vi "He3ReadOut_gpib.vi"(11 "reference":refnum<vi>) -> ()   [LabVIEW 2019]
uses:
  <vilib>/Utility/config.llb/Read Key (String).vi
  <vilib>/Utility/config.llb/NI_LVConfig.lvlib
panel:
  out "Last Updated":timestamp format="%<%Y-%m-%d %H:%M:%S>T"
  out "Device Version":dbl
  out "error out 4":errorcluster
  out "Pressure":waveform(dbl)[](graph)
  out "error out 3":errorcluster
  out "error out 2":errorcluster
  in  "Pressure":dbl caption="Torr"
  out "index":i32
  out "String 2":string
  out "error out":errorcluster
  out "String":string
  out "Status":bool
  out "Device Name":string
  in  "stop":bool
  out "data":string
  out "GPIB Address":string
  # "MKS Type 670 for He3 Pressure ReadOut"
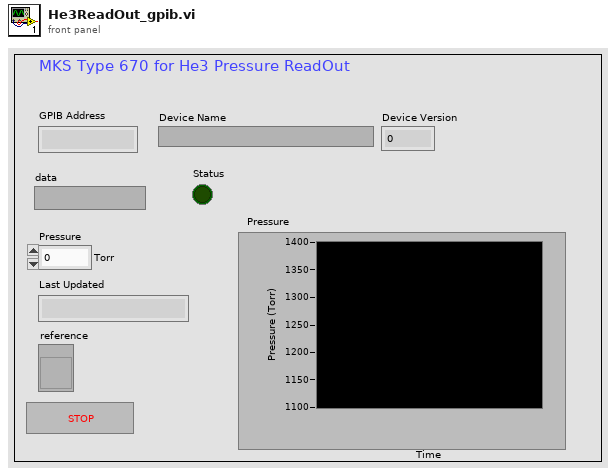
[diagram p1: front panel]
types:
  T1 = typedef "NI_LVConfig.lvlib/Config Data RefNum.ctl" = refnum<k1>
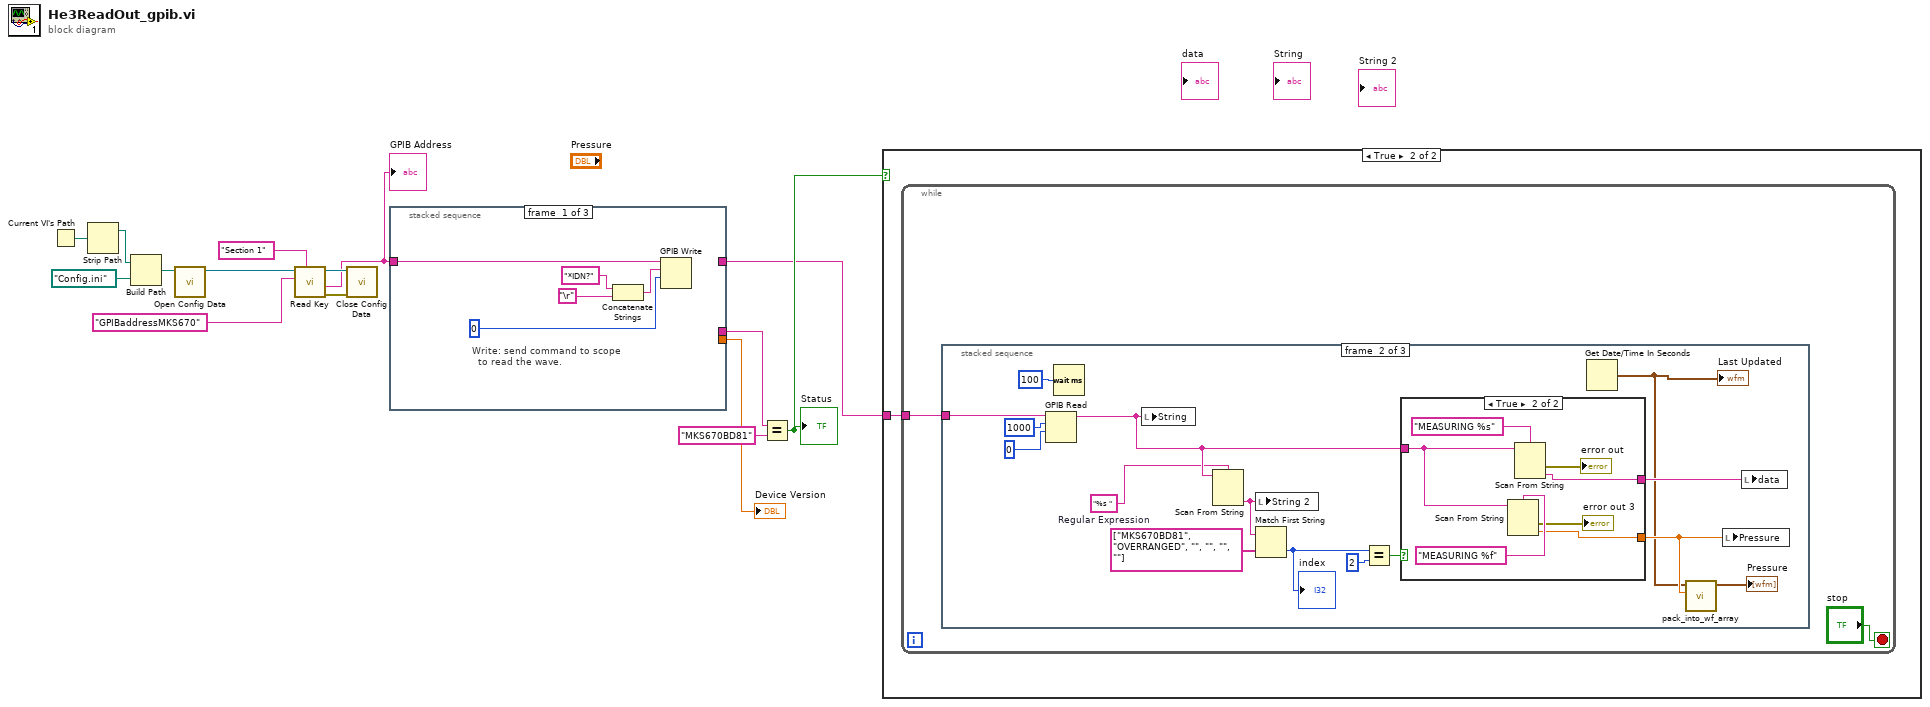
[diagram p0: block diagram]
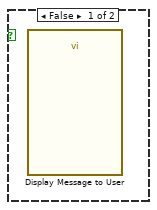
[diagram p2: hidden frame]
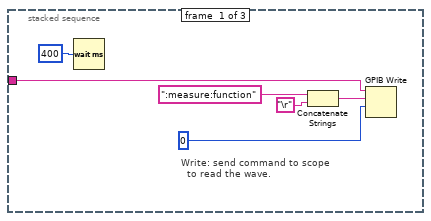
[diagram p3: hidden frame]
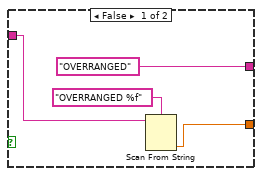
[diagram p4: hidden frame]
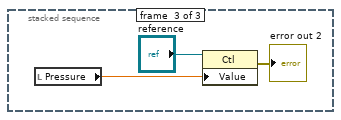
[diagram p5: hidden frame]
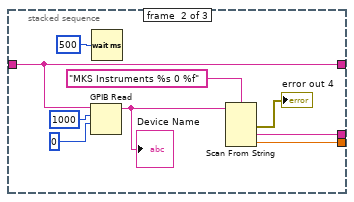
[diagram p6: hidden frame]
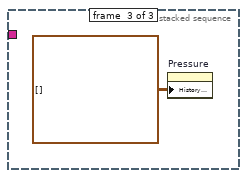
[diagram p7: hidden frame]
diagram:
  n1 = Current VI's Path() -> (path=w8:path)
  n2 = Strip Path(path=w8) -> (stripped path=w7:path)  [unwired: 1 out]
  n3 = Build Path(base path=w7, name or relative path=path "Config.ini" ("default name")) -> (appended path=w14:path)
  n4 = call <vilib>:"Open Config Data.vi"("configuration file path"=w14) -> ("refnum"=w9:T1)  [unwired: 8 in, 2 out]
  n5 = call-poly <vilib>:"Read Key.vi"("section"="Section 1", "key"="GPIBaddressMKS670", "refnum"=w9) -> ("error out"=w15:errorcluster, "value"=w6:string, "refnum out"=w11:T1)  [unwired: 5 in, 1 out]
  "GPIB Address" <- w6
  n6 = call <vilib>:"Close Config Data.vi"("error in (no error)"=w15, "refnum"=w11) -> ()  [unwired: 8 in, 2 out]
  n7 = stacked-sequence {
    tunnel: w6 -> [w16 w26 _]
    tunnel: [_ w26 _] -> w2
    tunnel: [_ w23 _] -> w5
    tunnel: [_ w21 _] -> w1
    frame #0 {
      # "Write: send command to scope\n  to read the wave."
      n8 = Concatenate Strings("*IDN?" ("data"), "\r") -> (w19:string)
      n9 = GPIB Write(0:w16, 1:w19, 2:0) -> ()  [unwired: 2 in, 2 out]
    }
    frame #1 {
      n10 = GPIB Read(0:w26, 1:1000 ("byte count"), 2:0) -> (5:w25:string)  [unwired: 2 in, 2 out]
      "Device Name" <- w25
      n11 = Wait (ms)(milliseconds to wait=u32 500) -> ()  [unwired: 1 out]
      n12 = Scan From String(format string="MKS Instruments %s 0 %f", input string=w25) -> (error out=→"error out 4":errorcluster, output 1=w23:string, output 2=w21:dbl)  [unwired: 4 in, 2 out]
    }
    frame #2 {
      n13 = property on="Pressure" class="WFChart (strict)"("History Data"=waveform(dbl)[][] []) -> ()  [unwired: 2 in, 2 out]
    }
  }
  "Device Version" <- w1
  n14 = Equal?(x=w5, y="MKS670BD81") -> (x = y?=w3:bool)
  "Status" <- w3
  n15 = case shown="True" w3 {
    tunnel: w2 -> [_ w31]
    frame False {
      n16 = call "Display Message to User"() -> ()  [unwired: 10 in, 2 out]
    }
    frame True {
      n17 = while {
        tunnel: w31 -> [w33]
        stop <- "stop" stop-if-true
        n18 = stacked-sequence {
          tunnel: w33 -> [w38 w53 _]
          frame #0 {
            # "Write: send command to scope\n  to read the wave."
            n19 = Wait (ms)(milliseconds to wait=u32 400) -> ()  [unwired: 1 out]
            n20 = Concatenate Strings(":measure:function" ("data"), "\r") -> (w37:string)
            n21 = GPIB Write(0:w38, 1:w37, 2:0) -> ()  [unwired: 2 in, 2 out]
          }
          frame #1 {
            w48 = "%s "  # Regular Expression
            n22 = GPIB Read(0:w53, 1:1000 ("byte count"), 2:0) -> (5:w49:string)  [unwired: 2 in, 2 out]
            n23 = Wait (ms)(milliseconds to wait=u32 100) -> ()  [unwired: 1 out]
            n24 = local write "String"(w49) -> ()
            n25 = Scan From String(format string=w48, input string=w49) -> (output 1=w44:string)  [unwired: 3 in, 3 out]
            n26 = local write "String 2"(w44) -> ()
            n27 = Match First String(2:string[] ["MKS670BD81", "OVERRANGED", "", "", "", ""], 3:w44) -> (0:w47:i32)  [unwired: 1 out]
            "index" <- w47
            n28 = Equal?(x=w47, y=2) -> (x = y?=w45:bool)
            n29 = case shown="True" w45 {
              tunnel: w49 -> [w58 w63]
              tunnel: ["OVERRANGED" ("data") w60] -> w43
              tunnel: [w55 w59] -> w41
              frame False {
                n30 = Scan From String(format string="OVERRANGED %f", input string=w58) -> (output 1=w55:dbl)  [unwired: 3 in, 3 out]
              }
              frame True {
                n31 = Scan From String(format string="MEASURING %f", input string=w63) -> (error out=→"error out 3":errorcluster, output 1=w59:dbl)  [unwired: 3 in, 2 out]
                n32 = Scan From String(format string="MEASURING %s", input string=w63) -> (error out=→"error out":errorcluster, output 1=w60:string)  [unwired: 3 in, 2 out]
              }
            }
            n33 = Get Date/Time In Seconds() -> (seconds since 1Jan1904=w40:timestamp)
            "Last Updated" <- w40
            n34 = call "pack_into_wf_array.vi"("pressure"=w41, "time"=w40) -> ("waveform_array"=→"Pressure":waveform(dbl)[])  [unwired: 9 in]
            n35 = local write "Pressure"(w41) -> ()
            n36 = local write "data"(w43) -> ()
          }
          frame #2 {
            n37 = local read "Pressure"() -> (w68:dbl)
            n38 = property class="Ctl"(reference="reference", "Value"=w68) -> (error out=→"error out 2":errorcluster)  [unwired: 1 in, 1 out]
          }
        }
      }
    }
  }
